vi "Acc.vi"() -> ()   [LabVIEW 2015]
doc: "The myRIO Project template acquires acceleration data from the onboard accelerometer and displays the changes of acceleration values in a waveform chart."
uses:
  <vilib>/myRIO/Instrument Drivers/Onboard IO/I2C/typedefs/I2C User Configuration.ctl
  <vilib>/myRIO/Instrument Drivers/Onboard IO/I2C/typedefs/I2C Transfer Rate.ctl
  <vilib>/Platform/TimedLoop/XDataNode/timing_clust.ctl
  <vilib>/Platform/TimedLoop/XDataNode/nitl_modes.ctl
  <vilib>/Platform/TimedLoop/XDataNode/wakeup.ctl
  <vilib>/myRIO/Common/Instrument Driver Framework/myRIO v1.0/UART/vis/myRIO v1.0 Close UART.vi
  <vilib>/Utility/error.llb/Error Cluster From Error Code.vi
  <vilib>/myRIO/Common/Instrument Driver Framework/myRIO v1.0/I2C/vis/myRIO v1.0 Configure I2C.vi
  <vilib>/myRIO/Common/Instrument Driver Framework/myRIO v1.0/I2C/vis/myRIO v1.0 Write I2C.vi
  <vilib>/myRIO/Common/Instrument Driver Framework/myRIO v1.0/I2C/vis/myRIO v1.0 Read I2C.vi
  <vilib>/myRIO/Common/Instrument Driver Framework/Utilities/vis/FPGA Ref Manager.vi
  <vilib>/myRIO/Common/Instrument Driver Framework/myRIO v1.0/myRIO v1.0 Reset FPGA.vi
  <vilib>/myRIO/Common/Instrument Driver Framework/myRIO v1.0/IRQ/vis/myRIO v1.0 IRQ Info FGV.vi
  <vilib>/myRIO/Common/Instrument Driver Framework/myRIO v1.0/IRQ/vis/myRIO v1.0 Timer IRQ Info FGV.vi
  <vilib>/myRIO/Common/Instrument Driver Framework/myRIO v1.0/IRQ/vis/myRIO v1.0 ISR Agent.vi
  <vilib>/platform/TimedLoop/XDataNode/XDataNode.xnode
  <vilib>/myRIO/Instrument Drivers/Utilities/Utilities.lvlib
  <vilib>/myRIO/Instrument Drivers/Onboard IO/I2C/I2C.lvlib
  <vilib>/Platform/TimedLoop/XDataNode/XDNodeRunTimeDep.lvlib
panel:
  out "Waveform Chart 2":cluster{dbl, dbl, dbl}(graph)
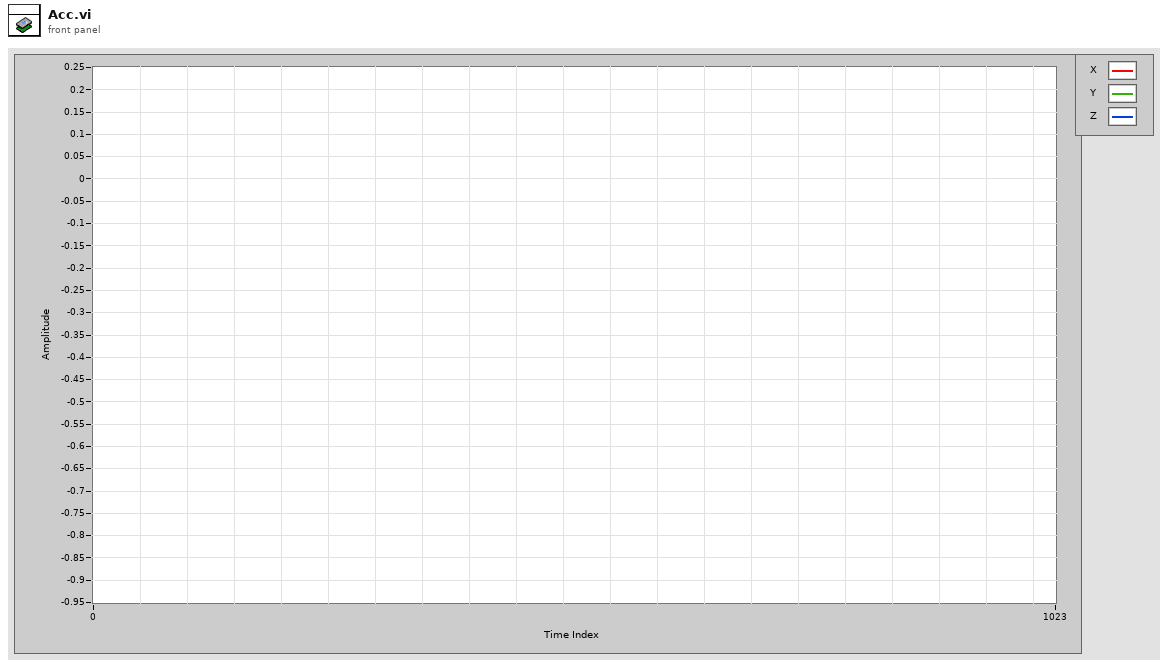
[diagram p1: front panel]
types:
  T1 = typedef "I2C.lvlib/I2C User Configuration.ctl" = cluster{"I2C Transfer Rate":T2}
  T2 = typedef "I2C.lvlib/I2C Transfer Rate.ctl" = enum16{"Standard mode (100 kbps)", "Fast mode (400 kbps)"}
  T3 = typedef "I2C.lvlib/I2C Reference.ctl" = cluster{"myRIO Reference":T4, "I2C Channels Enum":T8, "I2C Configuration":T9}
  T4 = typedef "myRIO Generic Hardware Reference.ctl" = cluster{"myRIO Model":T5, "myRIO Hardware Reference":T6}
  T5 = typedef "Hardware Version Enum.ctl" = enum16{"Unknown", "myRIO-1900", "myRIO-1950", "roboRIO"}
  T6 = typedef "myRIO v1.0 Reference.ctl" = cluster{"Generic FPGA Reference":T7, "Allow multiple opens":bool}
  T7 = typedef "Generic FPGA Reference.ctl" = refnum<k20>
  T8 = typedef "I2C Channels Enum.ctl" = enum16{"Not Connected", "A/I2C", "B/I2C", "I2C/I2C"}
  T9 = typedef "I2C.lvlib/I2C Configuration.ctl" = cluster{"I2C Transfer Rate":T2}
  T10 = typedef "XDNodeRunTimeDep.lvlib/timing_clust.ctl" = cluster{"Expected End [f-1]":u64, "Actual End [f-1]":u64, "Finished Late? [f-1]":bool, "Expected End [i-1]":u64, "Actual End [i-1]":u64, "Finished Late? [i-1]":bool, "Expected Start [i]":u64, "Actual Start [i]":u64, "Expected Start [f]":u64, "Actual Start [f]":u64, "Source Name":string, "Structure Name":string, "Period":i64, "Deadline":i64, "Offset":i64, "Start":i64, "Priority":i32, "Timeout":i32, "Mode":T11, "Wakeup Reason":T12, "Error":errorcluster, "Source Type":string, "Secondary Source Type":string, "Global End Time":u64, "Global Start Time":u64, "Frame Duration":u64, "Iteration Duration":u64, "Assigned CPU":i32, "I/O Scan Engine Mode":u32}
  T11 = typedef "XDNodeRunTimeDep.lvlib/nitl_modes.ctl" = enum32{"No Change", "Process missed periods, maintain original phase", "Discard missed periods, maintain original phase", "Process missed periods, ignore original phase", "Discard missed periods, ignore original phase"}
  T12 = typedef "XDNodeRunTimeDep.lvlib/wakeup.ctl" = enum32{"Normal", "Aborted", "Asynchronous wakeup", "Timing source error", "Timed loop error", "Timeout"}
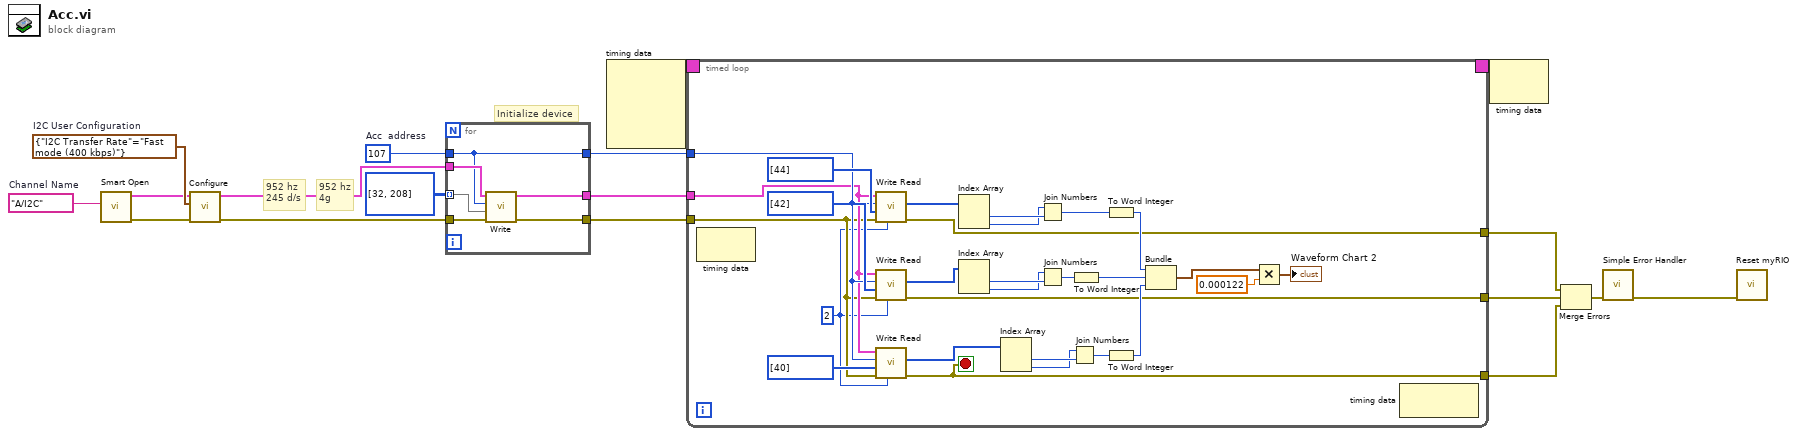
[diagram p0: block diagram]
diagram:
  w11 = u8 107  # Acc  address
  w16 = T1 {"I2C Transfer Rate"=enum."Fast mode (400 kbps)"}  # I2C User Configuration
  w17 = tag "A/I2C"  # Channel Name
  # "952 hz\n4g"
  # "952 hz\n245 d/s"
  # "Initialize device"
  n1 = call <vilib>:"Smart Open.vi"("Channel Name"=w17) -> ("error out"=w14:errorcluster, "I2C Ref Out"=w15:T3)  [unwired: 9 in]
  n2 = call <vilib>:"Configure.vi"("error in (no error)"=w14, "I2C User Configuration"=w16, "I2C Ref In"=w15) -> ("error out"=w7:errorcluster, "I2C Ref Out"=w8:T3)  [unwired: 7 in]
  n3 = for {
    tunnel: [w20] -> w6
    tunnel: [w19] -> w5
    tunnel: [w21] -> w10
    tunnel: u8[][] [[32, 208]] ("Bytes to Write") -> [w22] mode=indexing
    tunnel: w8 -> [w24]
    tunnel: w7 -> [w23]
    tunnel: w11 -> [w21]
    n4 = call <vilib>:"Write.vi"("error in (no error)"=w23, "Bytes to Write"=w22, "Slave Address (7-bit)"=w21, "I2C Ref In"=w24) -> ("error out"=w20:errorcluster, "I2C Ref Out"=w19:T3)  [unwired: 6 in]
  }
  n5 = node-c288() -> (w13:T10)  [unwired: 4 in]
  n6 = timed-loop {
    tunnel: [w42] -> w2
    timing: w13 -> [_]
    timing-out: [_] -> w12
    tunnel: w10 -> [w36]
    tunnel: w6 -> [w34]
    tunnel: w5 -> [w35]
    tunnel: [w33] -> w4
    tunnel: [w32] -> w3
    stop <- w42 stop-if-true
    w25 = u32 2 ("Byte Count")
    n7 = node-c288() -> ()  [unwired: 1 in, 1 out]
    n8 = call <vilib>:"Write Read.vi"("Byte Count"=w25, "error in (no error)"=w34, "Bytes to Write"=u8[] [44], "Slave Address (7-bit)"=w36, "I2C Ref In"=w35) -> ("error out"=w33:errorcluster, "Bytes Read"=w38:u8[])  [unwired: 3 in, 1 out]
    n9 = call <vilib>:"Write Read.vi"("Byte Count"=w25, "error in (no error)"=w34, "Bytes to Write"=u8[] [42], "Slave Address (7-bit)"=w36, "I2C Ref In"=w35) -> ("error out"=w32:errorcluster, "Bytes Read"=w40:u8[])  [unwired: 3 in, 1 out]
    n10 = call <vilib>:"Write Read.vi"("Byte Count"=w25, "error in (no error)"=w34, "Bytes to Write"=u8[] [40], "Slave Address (7-bit)"=w36, "I2C Ref In"=w35) -> ("error out"=w42:errorcluster, "Bytes Read"=w49:u8[])  [unwired: 3 in, 1 out]
    n11 = Index Array "Index Array"(array=w38) -> (element #1=w31:u8, element #2=w30:u8)  [unwired: 2 in]
    n12 = Index Array "Index Array"(array=w40) -> (element #1=w29:u8, element #2=w28:u8)  [unwired: 2 in]
    n13 = Index Array "Index Array"(array=w49) -> (element #1=w27:u8, element #2=w26:u8)  [unwired: 2 in]
    n14 = Join Numbers(hi=w30, lo=w31) -> ((hi.lo)=w52:u16)
    n15 = Join Numbers(hi=w28, lo=w29) -> ((hi.lo)=w51:u16)
    n16 = Join Numbers(hi=w26, lo=w27) -> ((hi.lo)=w50:u16)
    n17 = To Word Integer(number=w51) -> (16bit integer=w44:i16)
    n18 = To Word Integer(number=w52) -> (16bit integer=w45:i16)
    n19 = To Word Integer(number=w50) -> (16bit integer=w43:i16)
    n20 = Bundle "Bundle"(w45, w44, w43) -> (w47:cluster{i16, i16, i16})  [unwired: 1 in]
    n21 = Multiply(x=w47, y=0.000122) -> (x*y=→"Waveform Chart 2":cluster{dbl, dbl, dbl})
    n22 = node-c288() -> ()  [unwired: 1 in, 1 out]
  }
  n23 = node-c288(w12) -> ()  [unwired: 1 out]
  n24 = Merge Errors(w4, w3, w2) -> (w1:errorcluster)
  n25 = call <vilib>:"Simple Error Handler.vi"("error in (no error)"=w1) -> ("error out"=w18:errorcluster)  [unwired: 4 in, 4 out]
  n26 = call <vilib>:"Reset myRIO.vi"("error in (no error)"=w18) -> ()  [unwired: 10 in, 1 out]
